vi "Julian_project6.vi"() -> ()   [LabVIEW 2020]
uses:
  <vilib>/Instr/_visa.llb/VISA Configure Serial Port (Instr).vi
panel:
  out "array":string[][](array[string])
  out "read buffer 2":string
  out "Measurement 1":string
  out "read buffer":string
  in  "Combo Box 2":string(combo)
  in  "Combo Box":string(combo)
  out "Measurement 2":string
  in  "Set Function":bool
  out "Read Response 2":string
  in  "Delay Time (s) 2":dbl=0.5 format="%#_13g"
  in  "Measure":bool
  in  "VISA resource name":refnum<visa-resource-name>="COM3"
  in  "stop":bool
  # "VDC; -changes to volts dc\nVDC2;\nohms;\nohms2;\nVAC;\nVAC2;\nDIODE;\nDIODE2;\nFREQ;\nFREQ2;\n\nmeas1? -measures current mode\nmeas2? -measures 2 display"
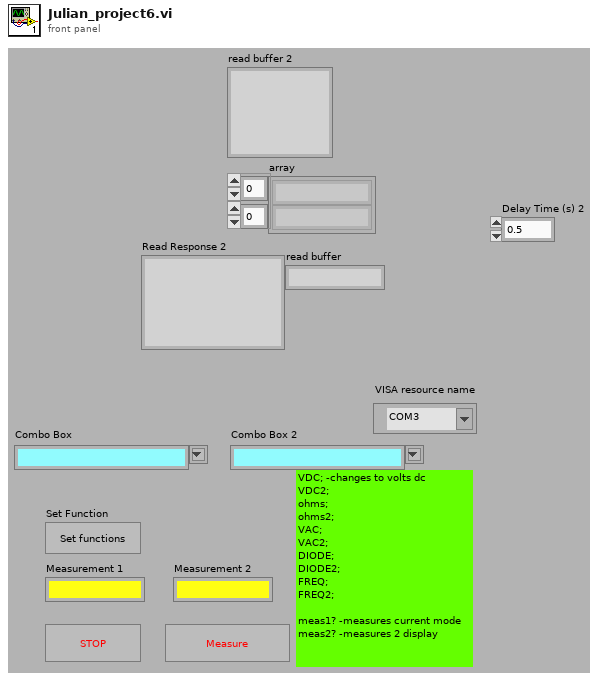
[diagram p1: front panel]
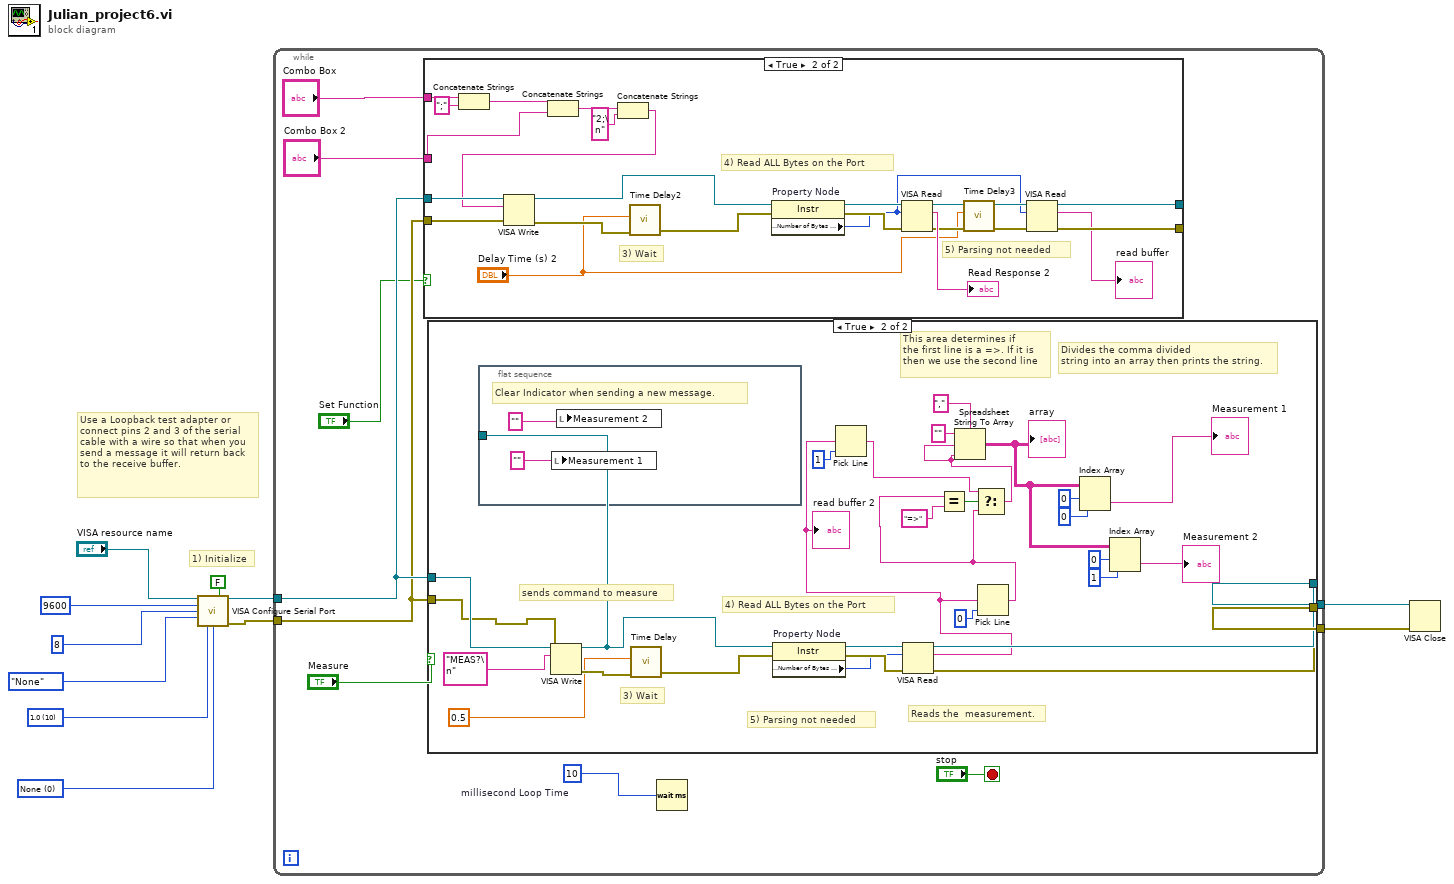
[diagram p0: block diagram]
diagram:
  w1 = u16 0 items=["None", "XON/XOFF", "RTS/CTS", "XON/XOFF & RTS/CTS", "DTR/DSR", "XON/XOFF & DTR/DSR"] ("Flow control")
  w2 = u16 10 items=["1.0"=10, "1.5"=15, "2.0"=20] ("Stop bits")
  # "Use a Loopback test adapter or connect pins 2 and 3 of the serial cable with a wire so that when you send a message it will return back to the receive buffer."
  # "1) Initialize"
  n1 = call-poly "VISA Configure Serial Port"("VISA resource name"="VISA resource name", "Enable Termination\nChar (T)"=FALSE ("Enable Termination\nChar (T)"), "baud rate (9600)"=u32 9600 ("Baud rate"), "data bits (8)"=u16 8 ("Data bits"), "parity (0:none)"=enum16{"None", "Odd", "Even", "Mark", "Space"}."None" ("Parity"), "stop bits (10: 1 bit)"=w2, "flow control (0:none)"=w1) -> ("VISA resource name out"=w10:refnum<visa-resource-name>, "error out"=w9:errorcluster)  [unwired: 1 in, 6 out]
  n2 = while {
    tunnel: w10 -> [w17]
    tunnel: w9 -> [w15]
    tunnel: [w16] -> w8
    tunnel: [w20] -> w7
    stop <- "stop" stop-if-true
    w18 = u32 10  # millisecond Loop Time
    n3 = case shown="True" "Set Function" {
      tunnel: w17 -> [w23 w46]
      tunnel: w15 -> [w22 w45]
      tunnel: [w23 w31] -> _
      tunnel: [w22 w30] -> _
      tunnel: "Combo Box" -> [_ w39]
      tunnel: "Combo Box 2" -> [_ w36]
      frame False {
      }
      frame True {
        # "5) Parsing not needed"
        # "3) Wait"
        # "4) Read ALL Bytes on the Port"
        n4 = Concatenate Strings(w39, ";" ("string")) -> (w37:string)
        n5 = Concatenate Strings(w37, w36) -> (w35:string)
        n6 = Concatenate Strings(w35, "2;\n" ("string")) -> (w33:string)
        n7 = VISA Write(VISA resource name=w46, write buffer=w33, error in (no error)=w45) -> (VISA resource name out=w40:refnum<visa-resource-name>, error out=w42:errorcluster)  [unwired: 1 out]
        n8 = call "Time Delay2"("error in (no error)"=w42, "Delay Time (s)"="Delay Time (s) 2") -> ("error out"=w41:errorcluster)  [unwired: 9 out]
        n9 = property on="Property Node" class="Instr"(reference=w40, error in=w41) -> (reference out=w44:refnum<visa-resource-name>, error out=w43:errorcluster, "Serial Settings:Number of Bytes at Serial Port"=w29:u32)
        n10 = VISA Read(VISA resource name=w44, byte count=w29, error in (no error)=w43) -> (VISA resource name out=w32:refnum<visa-resource-name>, read buffer=→"Read Response 2":string, error out=w26:errorcluster)  [unwired: 1 out]
        n11 = call "Time Delay3"("error in (no error)"=w26, "Delay Time (s)"="Delay Time (s) 2") -> ("error out"=w25:errorcluster)  [unwired: 9 out]
        n12 = VISA Read(VISA resource name=w32, byte count=w29, error in (no error)=w25) -> (VISA resource name out=w31:refnum<visa-resource-name>, read buffer=→"read buffer":string, error out=w30:errorcluster)  [unwired: 1 out]
      }
    }
    n13 = case shown="True" "Measure" {
      tunnel: w17 -> [w48 w73]
      tunnel: w15 -> [w47 w71]
      tunnel: [w48 w58] -> w16
      tunnel: [w47 w57] -> w20
      frame False {
      }
      frame True {
        # "Divides the comma divided \nstring into an array then prints the string."
        # "Reads the  measurement."
        # "sends command to measure"
        # "This area determines if \nthe first line is a =>. If it is\nthen we use the second line"
        # "5) Parsing not needed"
        # "3) Wait"
        # "4) Read ALL Bytes on the Port"
        n14 = flat-sequence {
          tunnel: w69 -> [_]
          frame #0 {
            # "Clear Indicator when sending a new message."
            n15 = local write "Measurement 1"("" ("Read Response")) -> ()
            n16 = local write "Measurement 2"("" ("Read Response")) -> ()
          }
        }
        n17 = VISA Write(VISA resource name=w73, write buffer="MEAS?\n" ("Sent Message"), error in (no error)=w71) -> (VISA resource name out=w69:refnum<visa-resource-name>, error out=w75:errorcluster)  [unwired: 1 out]
        n18 = call "Time Delay"("error in (no error)"=w75, "Delay Time (s)"=0.5) -> ("error out"=w74:errorcluster)  [unwired: 9 out]
        n19 = property on="Property Node" class="Instr"(reference=w69, error in=w74) -> (reference out=w77:refnum<visa-resource-name>, error out=w76:errorcluster, "Serial Settings:Number of Bytes at Serial Port"=w56:u32)
        n20 = VISA Read(VISA resource name=w77, byte count=w56, error in (no error)=w76) -> (VISA resource name out=w58:refnum<visa-resource-name>, read buffer=w51:string, error out=w57:errorcluster)  [unwired: 1 out]
        "read buffer 2" <- w51
        n21 = Pick Line(multi-line string=w51, line index=1) -> (output string=w50:string)  [unwired: 1 in]
        n22 = Pick Line(multi-line string=w51, line index=0) -> (output string=w54:string)  [unwired: 1 in]
        n23 = Equal?(x=w54, y="=>") -> (x = y?=w53:bool)
        n24 = Select(t=w50, s=w53, f=w54) -> (s? t:f=w49:string)
        n25 = Spreadsheet String To Array(delimiter (Tab)=",", format string="", spreadsheet string=w49, array type (2D Dbl)=w49) -> (array=w60:string[][])
        "array" <- w60
        n26 = Index Array(array=w60, index (row)=0, index (col)=0 ("disabled index (col)")) -> (element=→"Measurement 1":string)
        n27 = Index Array(array=w60, index (row)=0, index (col)=1 ("disabled index (col)")) -> (element=→"Measurement 2":string)
      }
    }
    n28 = Wait (ms)(milliseconds to wait=w18) -> ()  [unwired: 1 out]
  }
  n29 = VISA Close(VISA resource name=w8, error in (no error)=w7) -> ()  [unwired: 1 out]
